vi "Read File Data.vi"(8 "error in (no error)":errorcluster, 9 "Read Format (\"*n\")":string="\"*n\"", 10 "File Variable":string, 11 "VISA resource name":refnum<visa-resource-name>) -> (0 "error out":errorcluster, 2 "Read Data":string, 3 "VISA resource name out":refnum<visa-resource-name>)   [LabVIEW 2017, in "Keithley 2600 Series.lvlib"]
doc: "Reads data from a file."
uses:
  <instrlib>/Keithley 2600 Series/Keithley 2600 Series.lvlib
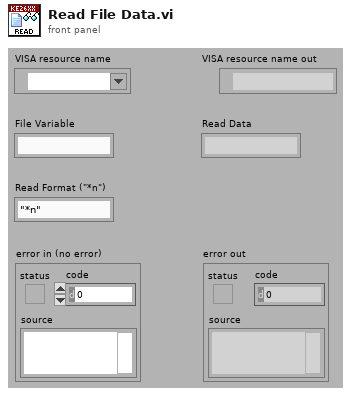
[diagram p1: front panel]
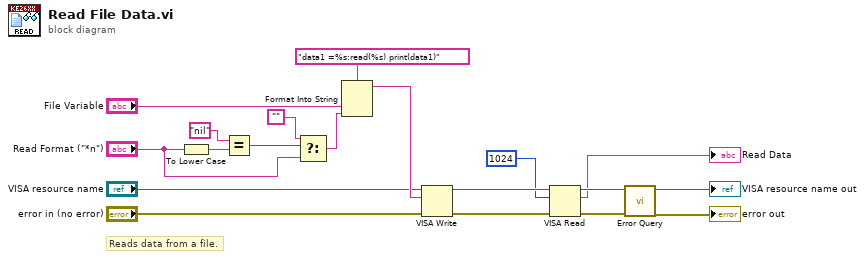
[diagram p0: block diagram]
diagram:
  # "Reads data from a file."
  n1 = To Lower Case(string="Read Format (\"*n\")") -> (all lower case string=w2:string)
  n2 = Equal?(x="nil", y=w2) -> (x = y?=w11:bool)
  n3 = Select(t="", s=w11, f="Read Format (\"*n\")") -> (s? t:f=w9:string)
  n4 = Format Into String(format string="data1 =%s:read(%s) print(data1)", "File Variable", w9) -> (resulting string=w18:string)  [unwired: 2 in, 1 out]
  n5 = VISA Write(VISA resource name="VISA resource name", write buffer=w18, error in (no error)="error in (no error)") -> (VISA resource name out=w8:refnum<visa-resource-name>, error out=w6:errorcluster)  [unwired: 1 out]
  n6 = VISA Read(VISA resource name=w8, byte count=u32 1024, error in (no error)=w6) -> (VISA resource name out=w7:refnum<visa-resource-name>, read buffer=→"Read Data":string, error out=w5:errorcluster)  [unwired: 1 out]
  n7 = call <instrlib>:"Error Query.vi"("error in (no error)"=w5, "VISA resource name"=w7) -> ("error out"=→"error out":errorcluster, "VISA resource name out"=→"VISA resource name out":refnum<visa-resource-name>)  [unwired: 6 in, 2 out]
